vi "Programacion paralela.vi"() -> ()   [LabVIEW 2020]
panel:
  out "Thermometer 9":u8(slide) scale=0.0..100.0
  out "Thermometer 8":u8(slide) scale=0.0..100.0
  out "Thermometer 7":u8(slide) scale=0.0..100.0
  out "Thermometer 6":u8(slide) scale=0.0..100.0
  out "Thermometer 5":u8(slide) scale=0.0..100.0
  out "Thermometer 4":u8(slide) scale=0.0..100.0
  out "Thermometer 3":u8(slide) scale=0.0..100.0
  out "Thermometer 2":u8(slide) scale=0.0..100.0
  out "Thermometer":u8(slide) scale=0.0..100.0
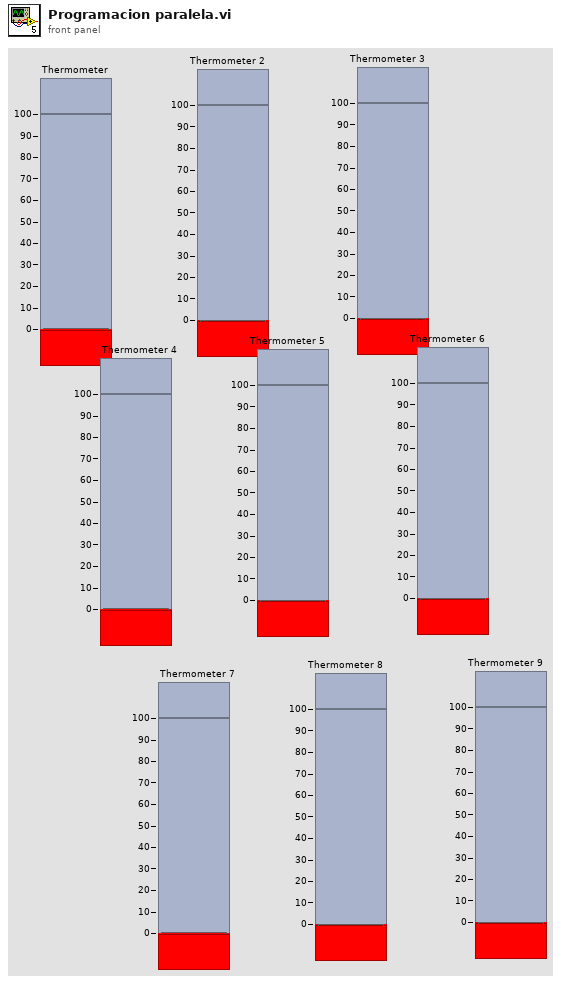
[diagram p1: front panel]
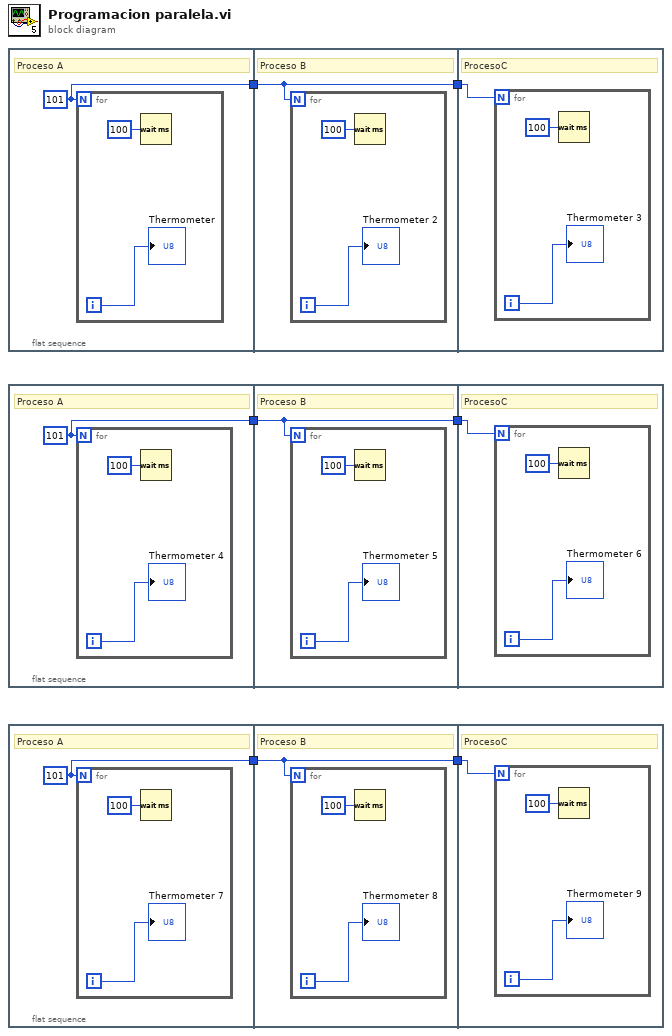
[diagram p0: block diagram]
diagram:
  n1 = flat-sequence {
    tunnel: [w7] -> w6
    tunnel: w6 -> [w10]
    tunnel: [w10] -> w5
    tunnel: w5 -> [w13]
    frame #0 {
      w7 = 101
      # "Proceso A"
      n2 = for {
        N: w7 -> [_]
        i -> [w8]
        n3 = Wait (ms)(milliseconds to wait=u32 100) -> ()  [unwired: 1 out]
        "Thermometer" <- w8
      }
    }
    frame #1 {
      # "Proceso B"
      n4 = for {
        N: w10 -> [_]
        i -> [w11]
        n5 = Wait (ms)(milliseconds to wait=u32 100) -> ()  [unwired: 1 out]
        "Thermometer 2" <- w11
      }
    }
    frame #2 {
      # "ProcesoC"
      n6 = for {
        N: w13 -> [_]
        i -> [w14]
        n7 = Wait (ms)(milliseconds to wait=u32 100) -> ()  [unwired: 1 out]
        "Thermometer 3" <- w14
      }
    }
  }
  n8 = flat-sequence {
    tunnel: [w16] -> w4
    tunnel: w4 -> [w19]
    tunnel: [w19] -> w3
    tunnel: w3 -> [w22]
    frame #0 {
      w16 = 101
      # "Proceso A"
      n9 = for {
        N: w16 -> [_]
        i -> [w17]
        n10 = Wait (ms)(milliseconds to wait=u32 100) -> ()  [unwired: 1 out]
        "Thermometer 4" <- w17
      }
    }
    frame #1 {
      # "Proceso B"
      n11 = for {
        N: w19 -> [_]
        i -> [w20]
        n12 = Wait (ms)(milliseconds to wait=u32 100) -> ()  [unwired: 1 out]
        "Thermometer 5" <- w20
      }
    }
    frame #2 {
      # "ProcesoC"
      n13 = for {
        N: w22 -> [_]
        i -> [w23]
        n14 = Wait (ms)(milliseconds to wait=u32 100) -> ()  [unwired: 1 out]
        "Thermometer 6" <- w23
      }
    }
  }
  n15 = flat-sequence {
    tunnel: [w25] -> w2
    tunnel: w2 -> [w28]
    tunnel: [w28] -> w1
    tunnel: w1 -> [w31]
    frame #0 {
      w25 = 101
      # "Proceso A"
      n16 = for {
        N: w25 -> [_]
        i -> [w26]
        n17 = Wait (ms)(milliseconds to wait=u32 100) -> ()  [unwired: 1 out]
        "Thermometer 7" <- w26
      }
    }
    frame #1 {
      # "Proceso B"
      n18 = for {
        N: w28 -> [_]
        i -> [w29]
        n19 = Wait (ms)(milliseconds to wait=u32 100) -> ()  [unwired: 1 out]
        "Thermometer 8" <- w29
      }
    }
    frame #2 {
      # "ProcesoC"
      n20 = for {
        N: w31 -> [_]
        i -> [w32]
        n21 = Wait (ms)(milliseconds to wait=u32 100) -> ()  [unwired: 1 out]
        "Thermometer 9" <- w32
      }
    }
  }
